vi "Case_Error.vi"() -> ()   [LabVIEW 2016]
panel:
  in  "Error In":errorcluster
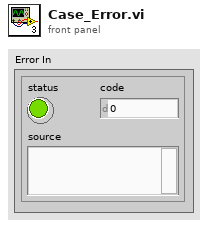
[diagram p1: front panel]
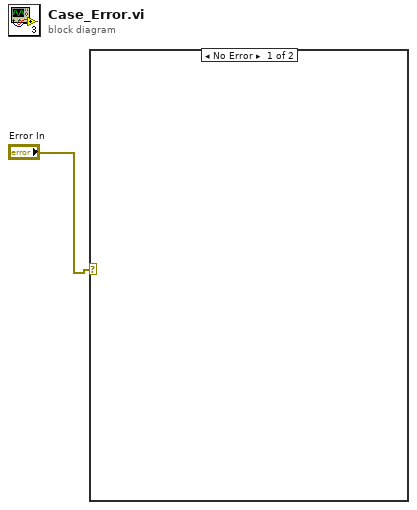
[diagram p0: block diagram]
diagram:
  n1 = case shown="No Error" "Error In" {
    frame No Error {
    }
    frame Error {
    }
  }
